vi "Handle TCP Connection.vi"(4 "Remote Port":u16, 6 "Remote Host":string, 7 "TCPMessageAPI":refnum<class "TCPMessageAPI.lvclass">, 8 "error in (no error)":errorcluster, 9 "Node ID":u32, 10 "Connection State":T1, 11 "RemoteMessagingHandler in":refnum<class "RemoteMessagingHandler.lvclass">) -> (0 "error out":errorcluster, 3 "RemoteMessagingHandler out":refnum<class "RemoteMessagingHandler.lvclass">)   [LabVIEW 2020, in "Volatus.lvlib" / "RemoteMessagingHandler.lvclass"]
uses:
  RemoteMessagingHandler.lvclass
  RemoteMessagingHandler.lvclass/RemoteMessagingHandler.ctl
  Event API/EventAPI.lvclass
  lv-vecto/Vecto/Connection State.ctl
  lv-vecto/Vecto/Vecto.lvlib
  lv-vecto/Vecto/TCPMessageService/TCPMessageAPI.lvclass
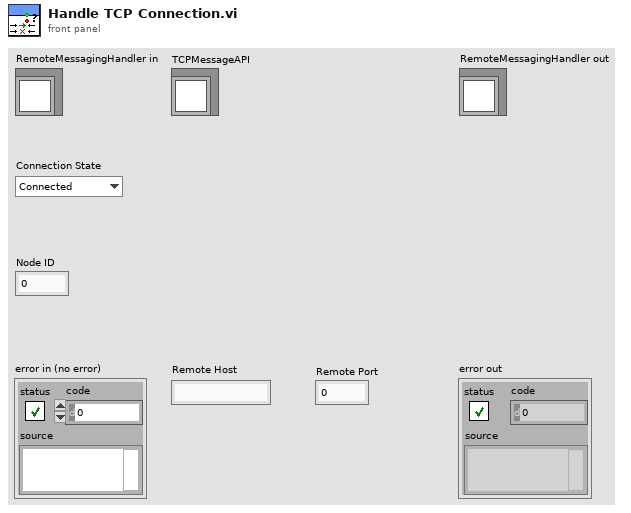
[diagram p1: front panel]
types:
  T1 = typedef "Vecto.lvlib/Connection State.ctl" = enum16{"Connected", "Disconnected"}
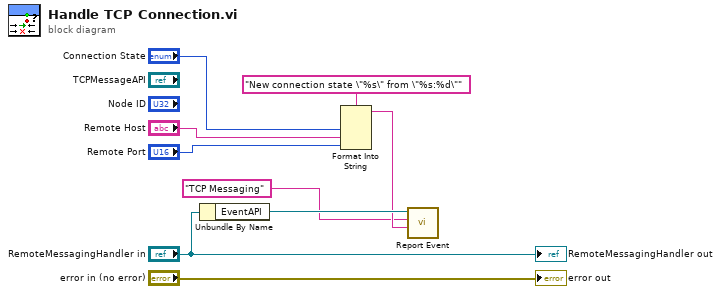
[diagram p0: block diagram]
diagram:
  n1 = Unbundle By Name("RemoteMessagingHandler in") -> ("EventAPI"=w3:refnum<class "EventAPI.lvclass">)
  n2 = Format Into String(format string="New connection state \"%s\" from \"%s:%d\"", "Connection State", "Remote Host", "Remote Port") -> (resulting string=w2:string)  [unwired: 2 in, 1 out]
  n3 = call "Report Event.vi"("Message"=w2, "Context"="TCP Messaging", "Event API in"=w3) -> ()  [unwired: 7 in, 2 out]
  "error out" <- "error in (no error)"
  "RemoteMessagingHandler out" <- "RemoteMessagingHandler in"
